vi "Path to User Data.vi"(8 "Error In":errorcluster) -> (0 "Error Out":errorcluster, 3 "Path To Run Time Support Folder":path)   [LabVIEW 2014]
uses:
  <vilib>/Utility/sysdir.llb/System Directory Type.ctl
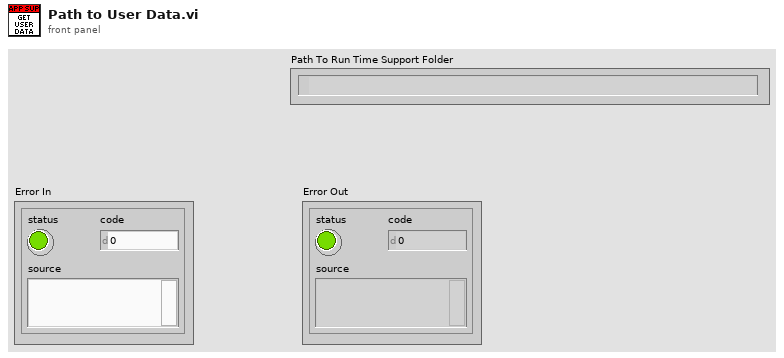
[diagram p1: front panel]
types:
  T1 = typedef "System Directory Type.ctl" = i32
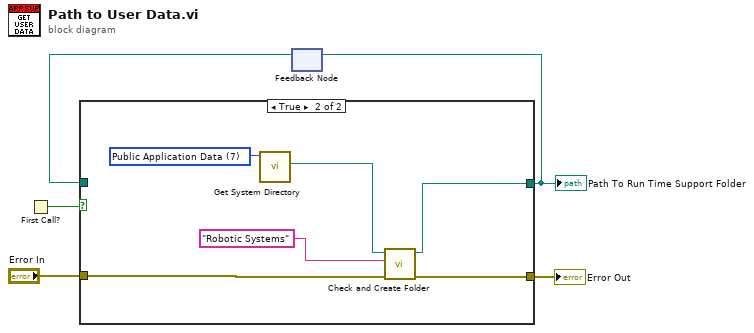
[diagram p0: block diagram]
diagram:
  n1 = First Call?() -> (First Call?: T/F=w5:bool)
  n2 = feedback #1() -> (w3:path)  [unwired: 1 in]
  n3 = case shown="True" w5 {
    tunnel: [w7 w12] -> w4
    tunnel: w3 -> [w7 _]
    tunnel: "Error In" -> [w6 w11]
    tunnel: [w6 w10] -> w1
    frame False {
    }
    frame True {
      w8 = T1 7 items=["User Home"=0, "User Desktop"=1, "User Documents"=2, "User Application Data"=3, "User Preferences"=4, "User Temporary"=5, "Public Documents"=6, "Public Application Data"=7, "Public Preferences"=8, "Public Cache"=13, "System Core Libraries"=9, "System Installed Libraries"=10, "Application Files"=11, "Boot Volume Root"=12] ("system directory type")
      n4 = call <vilib>:"Get System Directory.vi"("system directory type"=w8) -> ("system directory"=w9:path)  [unwired: 10 in]
      n5 = call "Check and Create Folder.vi"("error in"=w11, "Folder Name"="Robotic Systems" ("name or relative path"), "Path to Directory"=w9) -> ("error out"=w10:errorcluster, "Path to Folder"=w12:path)  [unwired: 7 in]
    }
  }
  "Path To Run Time Support Folder" <- w4
  "Error Out" <- w1
  n6 = feedback-in #1(w4) -> ()
